vi "sincosTest.vi"() -> ()   [LabVIEW 2015]
uses:
  <vilib>/rvi/FXPMathLib/FxpSinAndCos/subVIs/nifxpmath_SinAndCos_SimConfig.ctl
  <vilib>/Analysis/baseanly.llb/Mean (DBL).vi
  <vilib>/rvi/FXPMathLib/FxpSinAndCos/simVIs/DllFxpSinAndCosTemp_sub.vi
  <vilib>/rvi/FXPMathLib/FxpSinAndCos/XNode/nifxpmath_SinAndCos.xnode
  <vilib>/Analysis/NI_AALBase.lvlib
panel:
  out "CORDIC_sin_max":dbl
  out "CORDIC_cos_max":dbl
  out "CORDIC_sin_mean":dbl format="%0.5f"
  out "CORDIC_cos_mean":dbl format="%0.5f"
  out "CORDIC_sin_std":dbl format="%0.5f"
  out "CORDIC_cos_stddev":dbl format="%0.5f"
  out "sinsgl_stddev":dbl format="%0.5f"
  out "sinsgl_stddev":dbl format="%0.5f"
  out "sinfxp_stddev":dbl format="%0.5f"
  out "sinfxp_stddev":dbl format="%0.5f"
  out "cosfxp_mean":dbl format="%0.5f"
  out "sinfxp_mean":dbl format="%0.5f"
  out "cosfxp_max":dbl
  out "sinfxp_max":dbl
  out "stdcosfxp_mean":dbl format="%0.2f"
  out "stdsinfxp_mean":dbl format="%0.2f"
  out "stdcosfxp_max":dbl
  out "stdsinfxp_max":dbl
  out "cossgl_mean":dbl format="%0.5f"
  out "sinsgl_mean":dbl format="%0.5f"
  out "cossgl max":dbl
  out "sinsgl_max":dbl
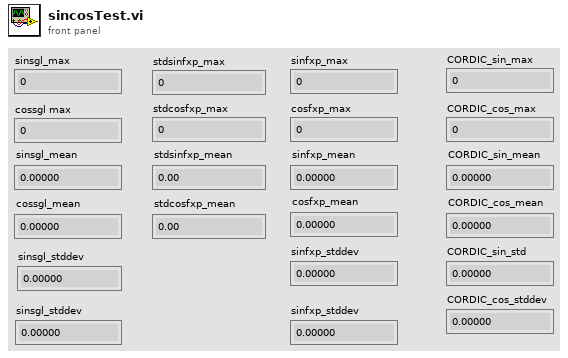
[diagram p1: front panel]
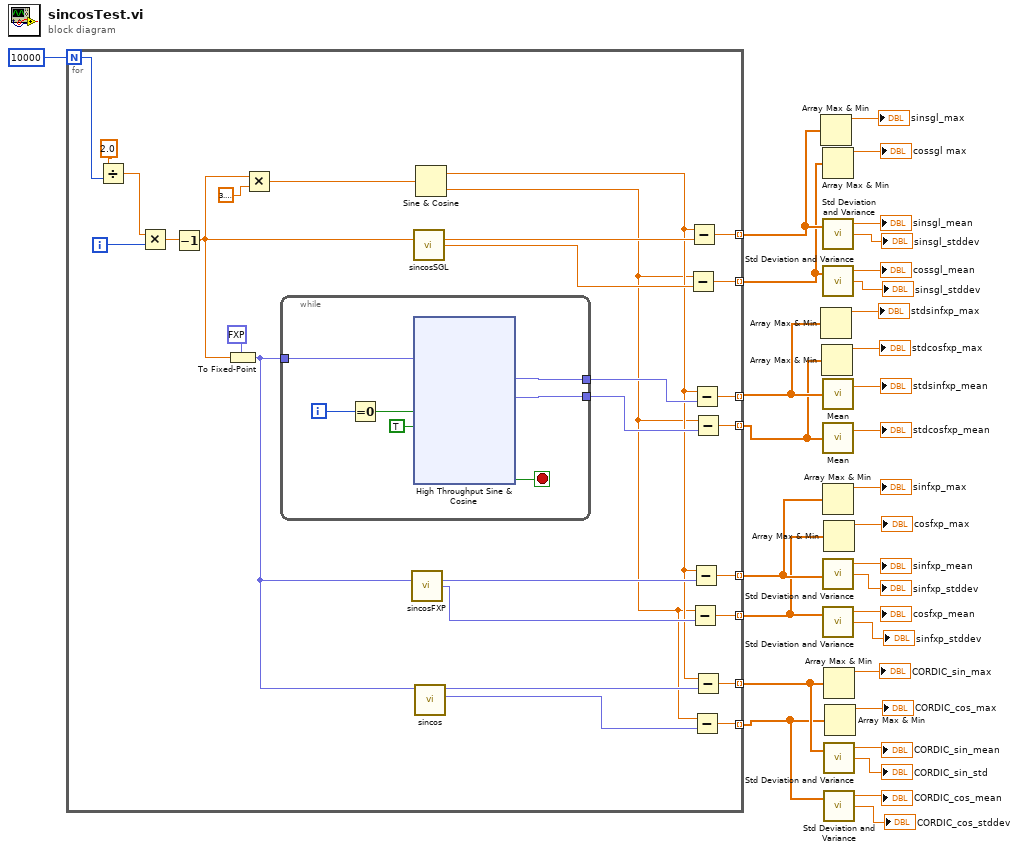
[diagram p0: block diagram]
diagram:
  n1 = for {
    N: 10000 -> [w44]
    tunnel: [w52] -> w30 mode=indexing
    tunnel: [w51] -> w29 mode=indexing
    tunnel: [w50] -> w28 mode=indexing
    tunnel: [w49] -> w27 mode=indexing
    tunnel: [w48] -> w26 mode=indexing
    tunnel: [w47] -> w25 mode=indexing
    tunnel: [w33] -> w3 mode=indexing
    tunnel: [w32] -> w2 mode=indexing
    i -> [w42]
    n2 = Divide(x=2.0 ("y"), y=w44) -> (x/y=w43:dbl)
    n3 = Multiply(x=w43, y=w42) -> (x*y=w41:dbl)
    n4 = Decrement(x=w41) -> (x-1=w40:dbl)
    n5 = To Fixed-Point(fixed-point type=fxp<+/-,16,1> 0.0 ("x (pi)"), number=w40) -> (fixed-point=w38:fxp<+/-,16,1>)
    n6 = Multiply(x=w40, y=3.141592653589793) -> (x*y=w39:dbl)
    n7 = while {
      tunnel: w38 -> [w66]
      tunnel: [w61] -> w55
      tunnel: [w60] -> w56
      i -> [w65]
      stop <- w62 stop-if-true
      n8 = Equal To 0?(x=w65) -> (x = 0?=w64:bool)
      n9 = xnode "High Throughput Sine & Cosine"("x (pi)"=w66, "input valid"=w64, "ready for output (T)"=TRUE) -> ("sin(x)"=w61:fxp<+/-,16,2>, "cos(x)"=w60:fxp<+/-,16,2>, "output valid"=w62:bool)  [unwired: 1 out]
    }
    n10 = call "sincosFXP.vi"("x"=w38) -> ("sinx"=w54:fxp<+/-,16,2>, "cosx"=w53:fxp<+/-,16,2>)  [unwired: 13 in]
    n11 = call "sincosSGL.vi"("x"=w40) -> ("sinx"=w58:sgl, "cosx"=w57:sgl)  [unwired: 13 in]
    n12 = call "sincos.vi"("x (pi)"=w38) -> ("cos(x)"=w34:fxp<+/-,16,2>, "sin(x)"=w37:fxp<+/-,16,2>)  [unwired: 9 in]
    n13 = Sine & Cosine(0:w39) -> (1:w36:dbl, 2:w35:dbl)
    n14 = Subtract(x=w35, y=w57) -> (x-y=w51:dbl)
    n15 = Subtract(x=w36, y=w58) -> (x-y=w52:dbl)
    n16 = Subtract(x=w35, y=w53) -> (x-y=w47:dbl)
    n17 = Subtract(x=w36, y=w54) -> (x-y=w48:dbl)
    n18 = Subtract(x=w36, y=w55) -> (x-y=w50:dbl)
    n19 = Subtract(x=w35, y=w34) -> (x-y=w32:dbl)
    n20 = Subtract(x=w35, y=w56) -> (x-y=w49:dbl)
    n21 = Subtract(x=w36, y=w37) -> (x-y=w33:dbl)
  }
  n22 = Array Max & Min(array=w30) -> (max value=→"sinsgl_max":dbl)  [unwired: 3 out]
  n23 = Array Max & Min(array=w28) -> (max value=→"stdsinfxp_max":dbl)  [unwired: 3 out]
  n24 = Array Max & Min(array=w27) -> (max value=→"stdcosfxp_max":dbl)  [unwired: 3 out]
  n25 = Array Max & Min(array=w29) -> (max value=→"cossgl max":dbl)  [unwired: 3 out]
  n26 = call <vilib>:"Std Deviation and Variance.vi"("X"=w30) -> ("mean"=→"sinsgl_mean":dbl, "standard deviation"=→"sinsgl_stddev":dbl)  [unwired: 1 in, 1 out]
  n27 = call <vilib>:"Std Deviation and Variance.vi"("X"=w29) -> ("mean"=→"cossgl_mean":dbl, "standard deviation"=→"sinsgl_stddev":dbl)  [unwired: 1 in, 1 out]
  n28 = call-poly <vilib>:"Mean.vi"("X"=w28) -> ("mean"=→"stdsinfxp_mean":dbl)  [unwired: 1 out]
  n29 = call-poly <vilib>:"Mean.vi"("X"=w27) -> ("mean"=→"stdcosfxp_mean":dbl)  [unwired: 1 out]
  n30 = Array Max & Min(array=w26) -> (max value=→"sinfxp_max":dbl)  [unwired: 3 out]
  n31 = call <vilib>:"Std Deviation and Variance.vi"("X"=w26) -> ("mean"=→"sinfxp_mean":dbl, "standard deviation"=→"sinfxp_stddev":dbl)  [unwired: 1 in, 1 out]
  n32 = call <vilib>:"Std Deviation and Variance.vi"("X"=w25) -> ("mean"=→"cosfxp_mean":dbl, "standard deviation"=→"sinfxp_stddev":dbl)  [unwired: 1 in, 1 out]
  n33 = Array Max & Min(array=w25) -> (max value=→"cosfxp_max":dbl)  [unwired: 3 out]
  n34 = Array Max & Min(array=w3) -> (max value=→"CORDIC_sin_max":dbl)  [unwired: 3 out]
  n35 = call <vilib>:"Std Deviation and Variance.vi"("X"=w3) -> ("mean"=→"CORDIC_sin_mean":dbl, "standard deviation"=→"CORDIC_sin_std":dbl)  [unwired: 1 in, 1 out]
  n36 = call <vilib>:"Std Deviation and Variance.vi"("X"=w2) -> ("mean"=→"CORDIC_cos_mean":dbl, "standard deviation"=→"CORDIC_cos_stddev":dbl)  [unwired: 1 in, 1 out]
  n37 = Array Max & Min(array=w2) -> (max value=→"CORDIC_cos_max":dbl)  [unwired: 3 out]
